vi "UE9 Frequency Measurement and Analog Input.vi"() -> ()   [LabVIEW 2021]
panel:
  in  "Case Constant\n(See Context Help)":bool=TRUE
  out "Iteration":i32
  out "Frequency (FIO2)":dbl format="%.2f"
  out "Period (FIO2)":dbl format="%.6f"
  in  "error in":errorcluster
  in  "ConnectionType":u16(ring) items=["LJ_ctUSB", "LJ_ctETHERNET"]
  in  "Address":string="1"
  in  "FirstFound":bool=TRUE
  in  "stop":bool
  out "FirmCounter (FIO1)":u32
  out "Counter0":u32
  out "error out":errorcluster
  out "Error Message":string
  out "AIN0-AIN7":dbl[](array[numeric]) format="%.6f"
  # "Timer clock is 320 kHz.  Assumes default high power level (Control firmware V1.08 or higher).\nFIO0 is 8-bit PWM output at 1250 Hz, with a 50% duty cycle.\nFIO1 is a firmware counter input.\nFIO2 is a 16-bit rising-to-rising edge measurement input.\nFIO3 is hardware counter 0.\nConnect jumpers from FIO0 to FIO1 to FIO2 to FIO3.  Or leave the jumper out of FIO0, and put an\nexternal signal into FIO1.\n\nShows that doing command/response analog input does not affect the timers and counters.\nEvery second, this VI measures the frequency of the 1250 Hz PWM output (using a hardware\ncounter, firmware counter, and edge-to-edge measurement), and then retrieves AIN0-AIN7\none hundred times."
  # "seconds"
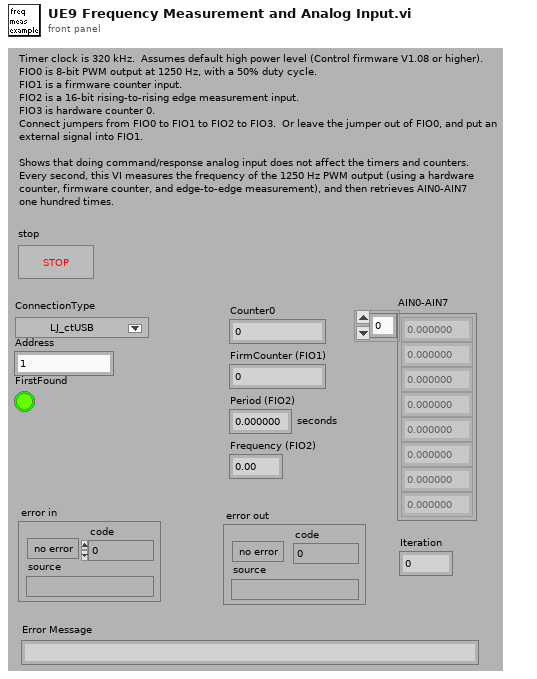
[diagram p1: front panel]
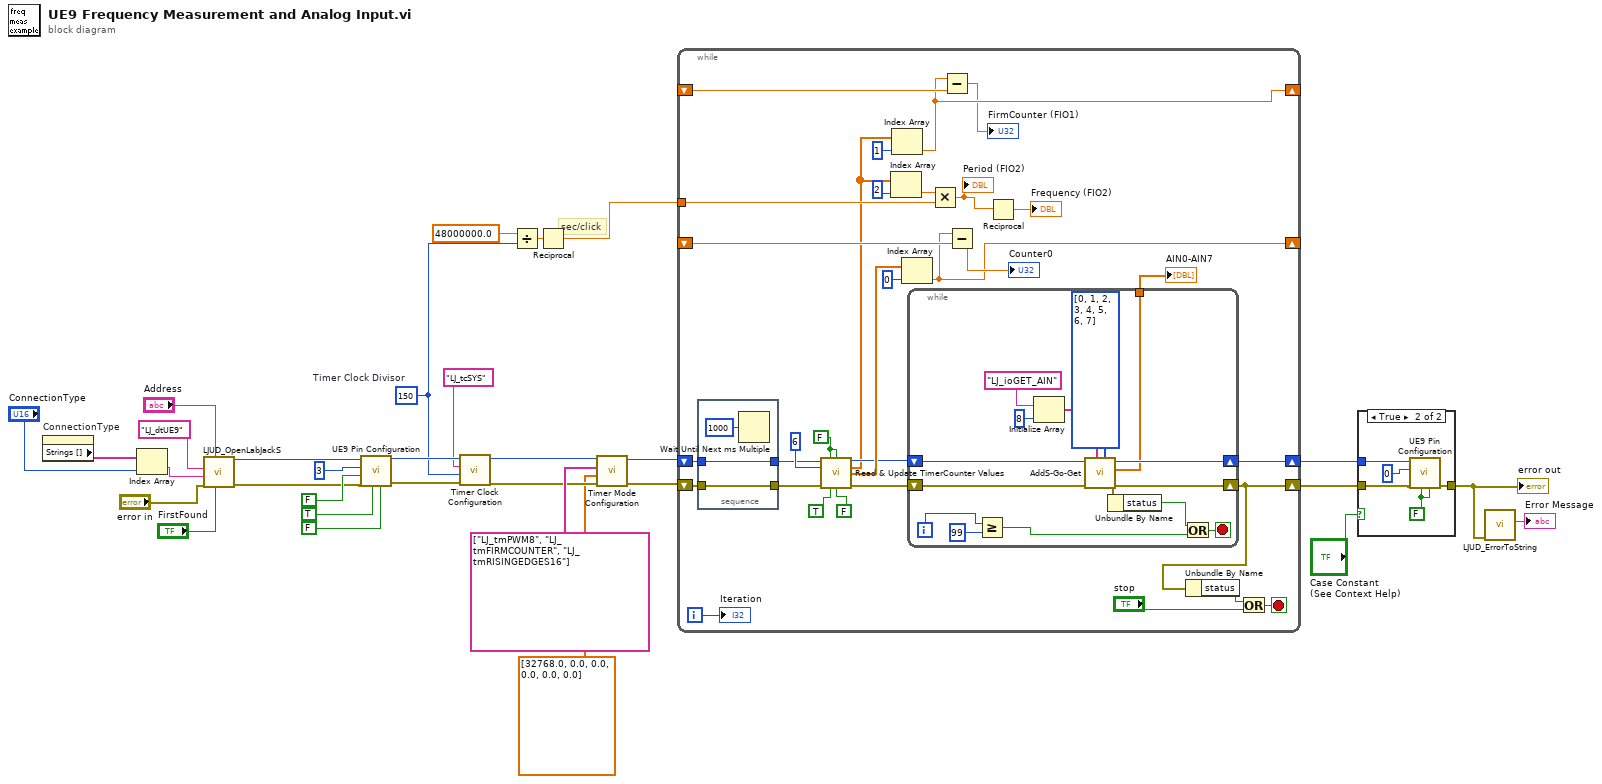
[diagram p0: block diagram]
diagram:
  w2 = 150  # Timer Clock Divisor
  # "sec/click"
  n1 = property on="ConnectionType" class="Ring (strict)"() -> ("Strings []"=w19:string[])  [unwired: 2 in, 2 out]
  n2 = Index Array(array=w19, index="ConnectionType") -> (element=w17:string)
  n3 = call "LJUD_OpenLabJackS.vi"("FirstFound"="FirstFound", "Address"="Address", "error in"="error in", "ConnectionType"=w17, "DeviceType"="LJ_dtUE9") -> ("error out"=w4:errorcluster, "Handle"=w3:i32)  [unwired: 4 in, 1 out]
  n4 = call "UE9 Pin Configuration.vi"("Enable Counter1"=FALSE ("Enable Counter0"), "Enable Counter0"=TRUE, "error in"=w4, "Enable DACs"=FALSE ("Enable Counter0"), "Number of Timers Enabled"=u8 3, "Handle In"=w3) -> ("error out"=w13:errorcluster, "Handle Out"=w12:i32)  [unwired: 4 in]
  n5 = call "Timer Clock Configuration.vi"("error in"=w13, "Timer Clock Divisor"=w2, "Timer Clock Base"="LJ_tcSYS", "Handle In"=w12) -> ("error out"=w14:errorcluster, "Handle Out"=w11:i32)  [unwired: 6 in]
  n6 = Divide(x=48000000.0, y=w2) -> (x/y=w22:dbl)
  n7 = Reciprocal(x=w22) -> (1/x=w21:dbl)
  n8 = call "Timer Mode Configuration.vi"("error in"=w14, "TimerValues"=dbl[] [32768.0, 0.0, 0.0, 0.0, 0.0, 0.0], "TimerModes"=string[] ["LJ_tmPWM8", "LJ_tmFIRMCOUNTER", "LJ_tmRISINGEDGES16"], "Handle In"=w11) -> ("error out"=w5:errorcluster, "Handle Out"=w6:i32)  [unwired: 6 in]
  n9 = while {
    shift-right: [w62] -> w27
    shift-left: w6 -> [w61]
    shift-right: [w48] -> w28
    shift-left: w5 -> [w60]
    tunnel: w21 -> [w46]
    shift-right: [w39] -> _
    shift-left: _ -> [w40]
    shift-right: [w41] -> _
    shift-left: _ -> [w43]
    i -> [w37]
    stop <- w50 stop-if-true
    w59 = FALSE ("Reset Counter0")
    n10 = stacked-sequence {
      tunnel: [w65] -> w53
      tunnel: [w64] -> w52
      tunnel: w61 -> [w65]
      tunnel: w60 -> [w64]
      frame #0 {
        n11 = Wait Until Next ms Multiple(millisecond multiple=u32 1000) -> ()  [unwired: 1 out]
      }
    }
    n12 = call "Read & Update TimerCounter Values.vi"("Handle In"=w53, "Reset Counter0"=w59, "Reset Counter1"=w59, "# Timers to Read"=6, "error in"=w52, "Read Counter0"=TRUE ("Reset Counter0"), "Read Counter1"=FALSE ("Reset Counter0")) -> ("Handle Out"=w54:i32, "Timer Value Reads"=w34:dbl[], "Counter Value Reads"=w57:dbl[], "error out"=w55:errorcluster)  [unwired: 5 in]
    n13 = Index Array(array=w34, index=2 ("Index")) -> (element=w35:dbl)
    n14 = Index Array(array=w34, index=1 ("Index")) -> (element=w39:dbl)
    n15 = Index Array(array=w57, index=0 ("Index")) -> (element=w41:dbl)
    n16 = while {
      shift-right: [w78] -> w62
      shift-left: w54 -> [w71]
      shift-right: [w77] -> w48
      shift-left: w55 -> [w79]
      tunnel: [w70] -> w63
      i -> [w74]
      stop <- w76 stop-if-true
      n17 = Greater Or Equal?(x=w74, y=99) -> (x >= y?=w72:bool)
      n18 = Initialize Array("LJ_ioGET_AIN" ("IOType"), 8 ("Dimension Size")) -> (w67:string[])
      n19 = call "AddS-Go-Get.vi"("Channels"=i32[] [0, 1, 2, 3, 4, 5, 6, 7], "IOTypes"=w67, "error in"=w79, "Handle In"=w71) -> ("error out"=w77:errorcluster, "Values Read"=w70:dbl[], "Handle Out"=w78:i32)  [unwired: 5 in]
      n20 = Unbundle By Name(w77) -> ("status"=w75:bool)
      n21 = Or(x=w75, y=w72) -> (x .or. y?=w76:bool)
    }
    "AIN0-AIN7" <- w63
    n22 = Multiply(x=w35, y=w46) -> (x*y=w45:dbl)
    "Period (FIO2)" <- w45
    n23 = Subtract(x=w39, y=w40) -> (x-y=→"FirmCounter (FIO1)":dbl)
    n24 = Subtract(x=w41, y=w43) -> (x-y=→"Counter0":dbl)
    n25 = Reciprocal(x=w45) -> (1/x=→"Frequency (FIO2)":dbl)
    n26 = Unbundle By Name(w48) -> ("status"=w49:bool)
    n27 = Or(x=w49, y="stop") -> (x .or. y?=w50:bool)
    "Iteration" <- w37
  }
  n28 = case shown="True" "Case Constant\n(See Context Help)" {
    tunnel: w28 -> [w81 w86]
    tunnel: w27 -> [_ w85]
    tunnel: [w81 w82] -> w30
    frame False {
    }
    frame True {
      w84 = FALSE ("Enable Counter0")
      n29 = call "UE9 Pin Configuration.vi"("Enable Counter1"=w84, "Enable Counter0"=w84, "error in"=w86, "Number of Timers Enabled"=u8 0 ("# Timers Enabled"), "Handle In"=w85) -> ("error out"=w82:errorcluster)  [unwired: 5 in, 1 out]
    }
  }
  "error out" <- w30
  n30 = call "LJUD_ErrorToString.vi"("error in"=w30) -> ("String"=→"Error Message":string)  [unwired: 10 in]
